vi "CleanUp.vi"(8 "error in (no error)":errorcluster, 11 "object in":refnum<class "SpectraPro.lvclass">) -> (0 "error out":errorcluster, 3 "object out":refnum<class "SpectraPro.lvclass">)   [LabVIEW 2019, in "SpectraPro.lvclass"]
uses:
  SpectraPro.lvclass
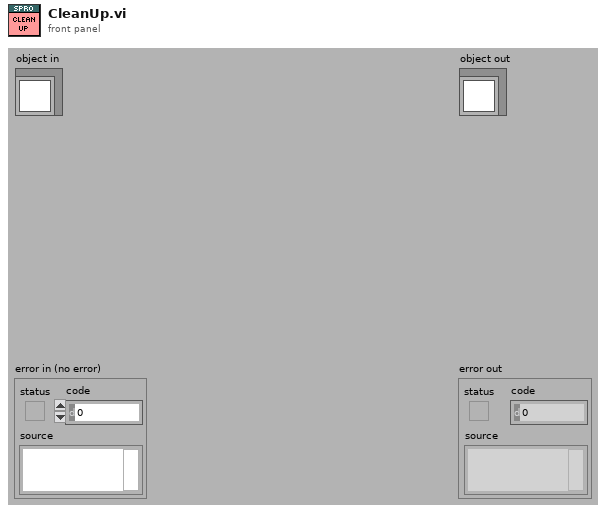
[diagram p1: front panel]
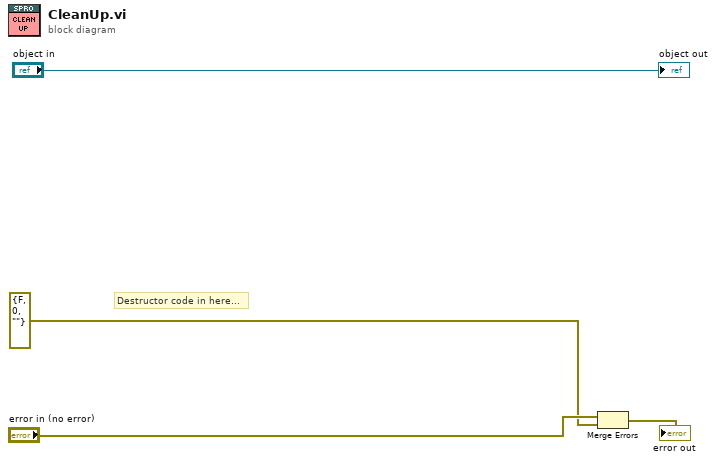
[diagram p0: block diagram]
diagram:
  # "Destructor code in here..."
  n1 = Merge Errors("error in (no error)", errorcluster {"status"=FALSE, "code"=0, "source"=""} ("error in (no error)")) -> (→"error out":errorcluster)
  "object out" <- "object in"
